vi "SeekReceipe_Local_Read_INI_Sub_VI.vi"(10 "Config File Path":path) -> (3 "Content from ini file":T1)   [LabVIEW 2017]
uses:
  <vilib>/Utility/config.llb/Read Key (I32).vi
  <vilib>/Utility/config.llb/Read Key (String).vi
  <vilib>/Utility/config.llb/Read Key (Path).vi
  <vilib>/Utility/config.llb/NI_LVConfig.lvlib
panel:
  # "Reads the parameter values from the ini file specified in below path"
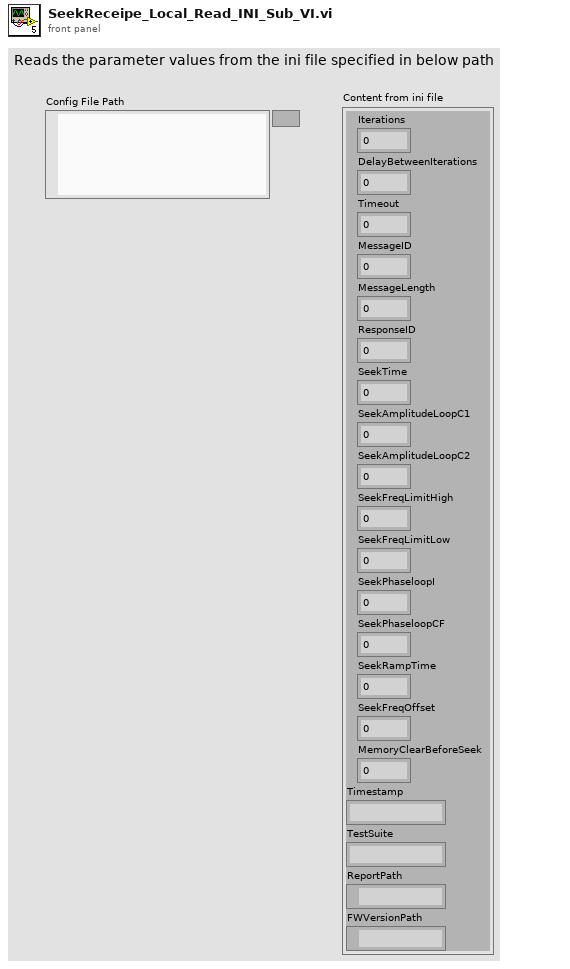
[diagram p1: front panel]
types:
  T1 = cluster{"Iterations":u64, "DelayBetweenIterations":u32, "Timeout":u32, "MessageID":i32, "MessageLength":i32, "ResponseID":i32, "SeekTime":i32, "SeekAmplitudeLoopC1":i32, "SeekAmplitudeLoopC2":i32, "SeekFreqLimitHigh":i32, "SeekFreqLimitLow":i32, "SeekPhaseloopI":i32, "SeekPhaseloopCF":i32, "SeekRampTime":i32, "SeekFreqOffset":i32, "MemoryClearBeforeSeek":i32, "Timestamp":string, "TestSuite":string, "ReportPath":path, "FWVersionPath":path}
  T2 = typedef "NI_LVConfig.lvlib/Config Data RefNum.ctl" = refnum<k1>
  T3 = cluster{u64, u32, u32, i32, i32, i32, i32, i32, i32, i32, i32, i32, i32, i32, i32, i32, "value":string, "value":string, "value":path, path}
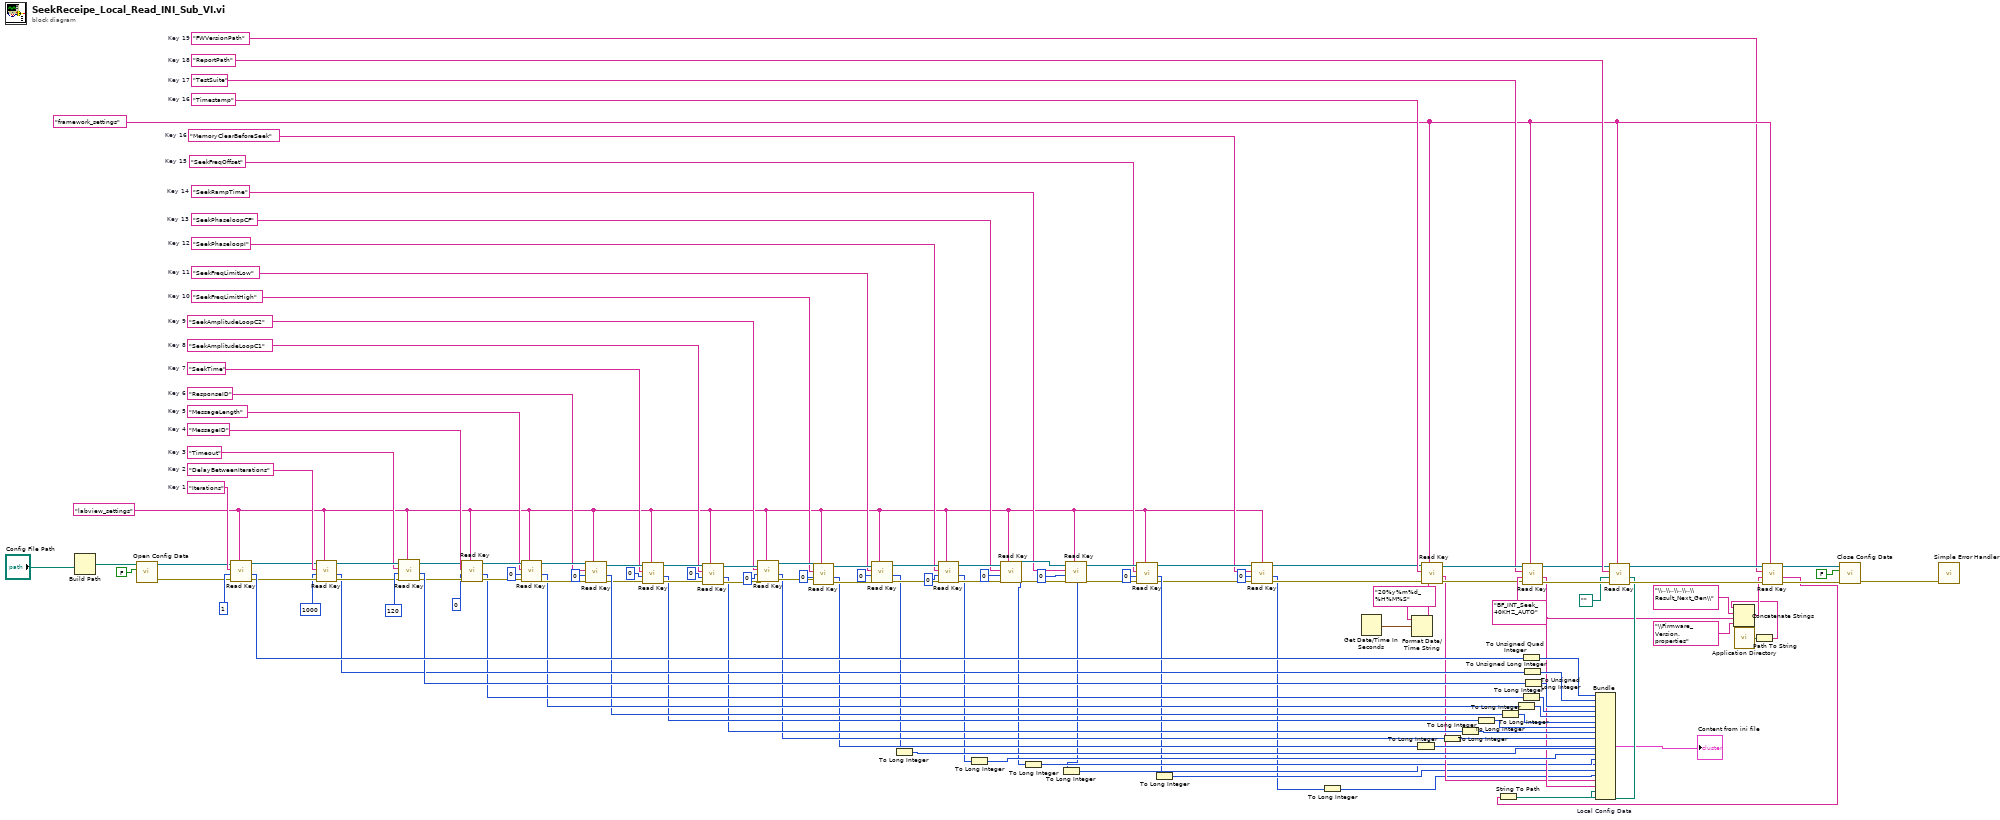
[diagram p0: block diagram]
diagram:
  w6 = "MemoryClearBeforeSeek"  # Key 16
  w21 = "SeekFreqOffset"  # Key 15
  w22 = "SeekRampTime"  # Key 14
  w23 = "SeekPhaseloopCF"  # Key 13
  w56 = "SeekPhaseloopI"  # Key 12
  w57 = "SeekFreqLimitLow"  # Key 11
  w58 = "SeekFreqLimitHigh"  # Key 10
  w11 = "SeekAmplitudeLoopC2"  # Key 9
  w59 = "SeekAmplitudeLoopC1"  # Key 8
  w60 = "SeekTime"  # Key 7
  w76 = "ResponseID"  # Key 6
  w77 = "MessageLength"  # Key 5
  w89 = "MessageID"  # Key 4
  w98 = "FWVersionPath"  # Key 19
  w110 = "Timestamp"  # Key 16
  w105 = "TestSuite"  # Key 17
  w111 = "Timeout"  # Key 3
  w120 = "ReportPath"  # Key 18
  w125 = "DelayBetweenIterations"  # Key 2
  w127 = "Iterations"  # Key 1
  w99 = "framework_settings" ("section")
  w5 = "labview_settings" ("section")
  n1 = Build Path(name or relative path="Config File Path") -> (appended path=w129:path)  [unwired: 1 in]
  n2 = call <vilib>:"Open Config Data.vi"("create file if necessary (T)"=FALSE ("create file if necessary? (T)"), "configuration file path"=w129) -> ("error out"=w92:errorcluster, "refnum"=w91:T2)  [unwired: 7 in, 1 out]
  n3 = call-poly <vilib>:"Read Key.vi"("section"=w5, "error in (no error)"=w92, "default value"=1, "key"=w127, "refnum"=w91) -> ("error out"=w123:errorcluster, "value"=w126:i32, "refnum out"=w124:T2)  [unwired: 4 out]
  n4 = call-poly <vilib>:"Read Key.vi"("section"=w5, "error in (no error)"=w123, "default value"=1000, "key"=w125, "refnum"=w124) -> ("error out"=w118:errorcluster, "value"=w90:i32, "refnum out"=w117:T2)  [unwired: 4 out]
  n5 = call-poly <vilib>:"Read Key.vi"("section"=w5, "error in (no error)"=w118, "default value"=120, "key"=w111, "refnum"=w117) -> ("error out"=w85:errorcluster, "value"=w115:i32, "refnum out"=w88:T2)  [unwired: 4 out]
  n6 = call-poly <vilib>:"Read Key.vi"("section"=w5, "error in (no error)"=w85, "default value"=0, "key"=w89, "refnum"=w88) -> ("error out"=w83:errorcluster, "value"=w82:i32, "refnum out"=w87:T2)  [unwired: 4 out]
  n7 = call-poly <vilib>:"Read Key.vi"("section"=w5, "error in (no error)"=w83, "default value"=0, "key"=w77, "refnum"=w87) -> ("error out"=w84:errorcluster, "value"=w79:i32, "refnum out"=w86:T2)  [unwired: 4 out]
  n8 = call-poly <vilib>:"Read Key.vi"("section"=w5, "error in (no error)"=w84, "default value"=0, "key"=w76, "refnum"=w86) -> ("error out"=w55:errorcluster, "value"=w78:i32, "refnum out"=w66:T2)  [unwired: 4 out]
  n9 = call-poly <vilib>:"Read Key.vi"("section"=w5, "error in (no error)"=w55, "default value"=0, "key"=w60, "refnum"=w66) -> ("error out"=w51:errorcluster, "value"=w46:i32, "refnum out"=w65:T2)  [unwired: 4 out]
  n10 = call-poly <vilib>:"Read Key.vi"("section"=w5, "error in (no error)"=w51, "default value"=0, "key"=w59, "refnum"=w65) -> ("error out"=w54:errorcluster, "value"=w44:i32, "refnum out"=w64:T2)  [unwired: 4 out]
  n11 = call-poly <vilib>:"Read Key.vi"("section"=w5, "error in (no error)"=w54, "default value"=0, "key"=w11, "refnum"=w64) -> ("error out"=w53:errorcluster, "value"=w42:i32, "refnum out"=w63:T2)  [unwired: 4 out]
  n12 = call-poly <vilib>:"Read Key.vi"("section"=w5, "error in (no error)"=w53, "default value"=0, "key"=w58, "refnum"=w63) -> ("error out"=w50:errorcluster, "value"=w40:i32, "refnum out"=w62:T2)  [unwired: 4 out]
  n13 = call-poly <vilib>:"Read Key.vi"("section"=w5, "error in (no error)"=w50, "default value"=0, "key"=w57, "refnum"=w62) -> ("error out"=w52:errorcluster, "value"=w38:i32, "refnum out"=w61:T2)  [unwired: 4 out]
  n14 = To Long Integer(number=w38) -> (32bit integer=w37:i32)
  n15 = call-poly <vilib>:"Read Key.vi"("section"=w5, "error in (no error)"=w52, "default value"=0, "key"=w56, "refnum"=w61) -> ("error out"=w35:errorcluster, "value"=w34:i32, "refnum out"=w33:T2)  [unwired: 4 out]
  n16 = To Long Integer(number=w34) -> (32bit integer=w36:i32)
  n17 = call-poly <vilib>:"Read Key.vi"("section"=w5, "error in (no error)"=w35, "default value"=0, "key"=w23, "refnum"=w33) -> ("error out"=w29:errorcluster, "value"=w17:i32, "refnum out"=w32:T2)  [unwired: 4 out]
  n18 = To Long Integer(number=w17) -> (32bit integer=w16:i32)
  n19 = call-poly <vilib>:"Read Key.vi"("section"=w5, "error in (no error)"=w29, "default value"=0, "key"=w22, "refnum"=w32) -> ("error out"=w30:errorcluster, "value"=w15:i32, "refnum out"=w31:T2)  [unwired: 4 out]
  n20 = To Long Integer(number=w15) -> (32bit integer=w14:i32)
  n21 = call-poly <vilib>:"Read Key.vi"("section"=w5, "error in (no error)"=w30, "default value"=0, "key"=w21, "refnum"=w31) -> ("error out"=w8:errorcluster, "value"=w13:i32, "refnum out"=w10:T2)  [unwired: 4 out]
  n22 = To Long Integer(number=w13) -> (32bit integer=w12:i32)
  n23 = call-poly <vilib>:"Read Key.vi"("section"=w5, "error in (no error)"=w8, "default value"=0, "key"=w6, "refnum"=w10) -> ("error out"=w7:errorcluster, "value"=w3:i32, "refnum out"=w9:T2)  [unwired: 4 out]
  n24 = To Long Integer(number=w3) -> (32bit integer=w2:i32)
  n25 = Get Date/Time In Seconds() -> (seconds since 1Jan1904=w112:timestamp)
  n26 = Format Date/Time String(time format string (%c)="20%y%m%d_%H%M%S", seconds (now)=w112) -> (date/time string=w113:string)  [unwired: 1 out]
  n27 = To Long Integer(number=w40) -> (32bit integer=w39:i32)
  n28 = call-poly <vilib>:"Read Key.vi"("section"=w99, "error in (no error)"=w7, "default value"=w113, "key"=w110, "refnum"=w9) -> ("error out"=w107:errorcluster, "value"=w24:string, "refnum out"=w108:T2)  [unwired: 1 in, 3 out]
  n29 = To Long Integer(number=w42) -> (32bit integer=w41:i32)
  n30 = To Long Integer(number=w44) -> (32bit integer=w43:i32)
  n31 = To Long Integer(number=w46) -> (32bit integer=w45:i32)
  n32 = To Long Integer(number=w78) -> (32bit integer=w49:i32)
  n33 = To Long Integer(number=w79) -> (32bit integer=w80:i32)
  n34 = To Unsigned Quad Integer(1:w126) -> (0:w133:u64)
  n35 = To Long Integer(number=w82) -> (32bit integer=w81:i32)
  n36 = call-poly <vilib>:"Read Key.vi"("section"=w99, "error in (no error)"=w107, "default value"="BF_INT_Seek_40KHZ_AUTO", "key"=w105, "refnum"=w108) -> ("error out"=w106:errorcluster, "value"=w25:string, "refnum out"=w109:T2)  [unwired: 1 in, 3 out]
  n37 = To Unsigned Long Integer(number=w90) -> (unsigned 32bit integer=w48:u32)
  n38 = To Unsigned Long Integer(number=w115) -> (unsigned 32bit integer=w47:u32)
  n39 = call-poly <vilib>:"Read Key.vi"("section"=w99, "error in (no error)"=w106, "default value"=path "", "key"=w120, "refnum"=w109) -> ("error out"=w100:errorcluster, "value"=w26:path, "refnum out"=w103:T2)  [unwired: 1 in, 3 out]
  n40 = call <vilib>:"Application Directory.vi"() -> ("Application Directory"=w94:path)
  n41 = Path To String(path=w94) -> (string=w93:string)
  n42 = Concatenate Strings(w93, "\\..\\..\\..\\..\\Result_Next_Gen\\" ("default value"), w25, "\\Firmware_Version.properties" ("default value")) -> (w97:string)
  n43 = call-poly <vilib>:"Read Key.vi"("section"=w99, "error in (no error)"=w100, "default value"=w97, "key"=w98, "refnum"=w103) -> ("error out"=w101:errorcluster, "value"=w28:string, "refnum out"=w102:T2)  [unwired: 1 in, 3 out]
  n44 = String To Path(string=w28) -> (path=w27:path)
  n45 = Bundle "Local Config Data"(w133, w48, w47, w81, w80, w49, w45, w43, w41, w39, w37, w36, w16, w14, w12, w2, "value"=w24, "value"=w25, "value"=w26, w27) -> (→"Content from ini file":T3)  [unwired: 1 in]
  n46 = call <vilib>:"Close Config Data.vi"("error in (no error)"=w101, "write file if changed (T)"=FALSE ("write configuration file? (T)"), "refnum"=w102) -> ("error out"=w130:errorcluster)  [unwired: 8 out]
  n47 = call <vilib>:"Simple Error Handler.vi"("error in (no error)"=w130) -> ()  [unwired: 1 in, 8 out]
